vi "TCPListener.vi"(7 "stop":bool, 11 "port":u16=16240) -> ()   [LabVIEW 2026]
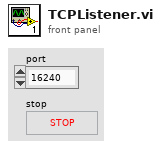
[diagram p1: front panel]
types:
  T1 = cluster{"peripheral":string, "function":string, "args":string}
  T2 = enum16{"Standard", "Buffered", "CRLF", "Immediate"}
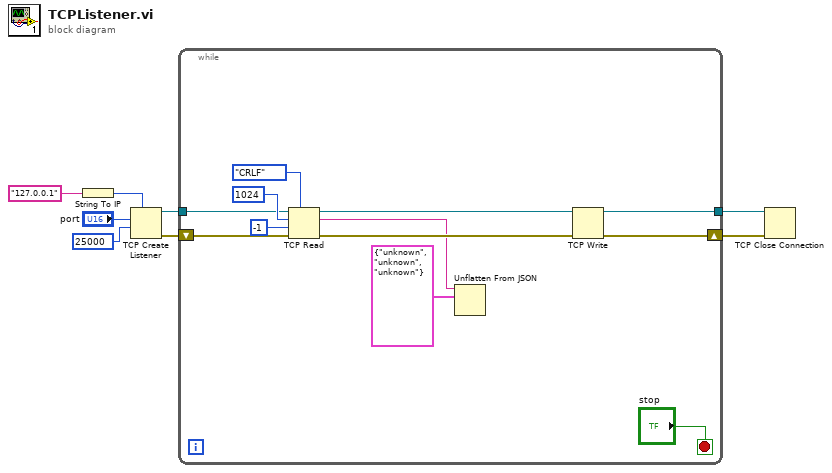
[diagram p0: block diagram]
diagram:
  n1 = String To IP(1:"127.0.0.1" ("address")) -> (0:w6:u32)
  n2 = TCP Create Listener(7:w6, 9:25000 ("timeout ms (25000)"), 10:"port") -> (0:w1:errorcluster, 3:w4:refnum<k5>)  [unwired: 2 in, 1 out]
  n3 = while {
    tunnel: w4 -> [w16]
    tunnel: [w14] -> w3
    shift-right: [w12] -> w2
    shift-left: w1 -> [w11]
    stop <- "stop" stop-if-true
    n4 = TCP Read(connection ID=w16, bytes to read=1024, error in (no error)=w11, 7:T2."CRLF" ("mode (standard)"), 9:-1 ("timeout ms (25000)")) -> (connection ID out=w15:refnum<k5>, data out=w10:string, error out=w13:errorcluster)
    n5 = Unflatten From JSON(JSON string=w10, type and defaults=T1 {"peripheral"="unknown", "function"="unknown", "args"="unknown"}) -> ()  [unwired: 5 in, 2 out]
    n6 = TCP Write(connection ID=w15, error in (no error)=w13) -> (connection ID out=w14:refnum<k5>, error out=w12:errorcluster)  [unwired: 2 in, 1 out]
  }
  n7 = TCP Close Connection(connection ID=w3, error in (no error)=w2) -> ()  [unwired: 1 in, 2 out]
